vi "weather_station.vi"() -> ()   [LabVIEW 2023]
uses:
  <vilib>/Instr/_visa.llb/VISA Configure Serial Port (Instr).vi
  global_variables.vi
  <vilib>/addons/_JKI.lib/REST Client/classes/REST Client/REST Client.lvclass
  <vilib>/Analysis/NI_AALBase.lvlib
panel:
  in  "stop_button":bool
  in  "HELP_BUTTON":bool
  in  "SAVE DATA":bool
  in  "COUNT SERVER":i8 min=0
  in  "REQUEST_TO_SERVER":bool
  in  "LOAD_FROM_FILE":bool
  in  "PLAY_STOP_BUTTON":bool
  in  "ACQUISITION TIME":dbl min=0.0
  out "?":bool
  out "?":bool
  out "?":bool
  out "?":bool
  in  "VISA RESOURCE NAME":refnum<visa-resource-name>
  out "?":string[](array[string])
  out "?":string[](array[string])
  out "?":string[](array[string])
  out "HUMIDITY":dbl(knob) scale=0.0..100.0
  out "PERCEIVED TEMP.":dbl(slide) scale=0.0..100.0
  out "TEMPERATURE":dbl(slide) scale=0.0..100.0
  out "HUMIDITY TREND":cluster{dbl, dbl}(graph)
  out "PERCEIVED TEMP. TREND":cluster{dbl, dbl}(graph)
  out "TEMPERATURE TREND":cluster{dbl, dbl}(graph)
  # "ACQUISITION FROM ARDUINO"
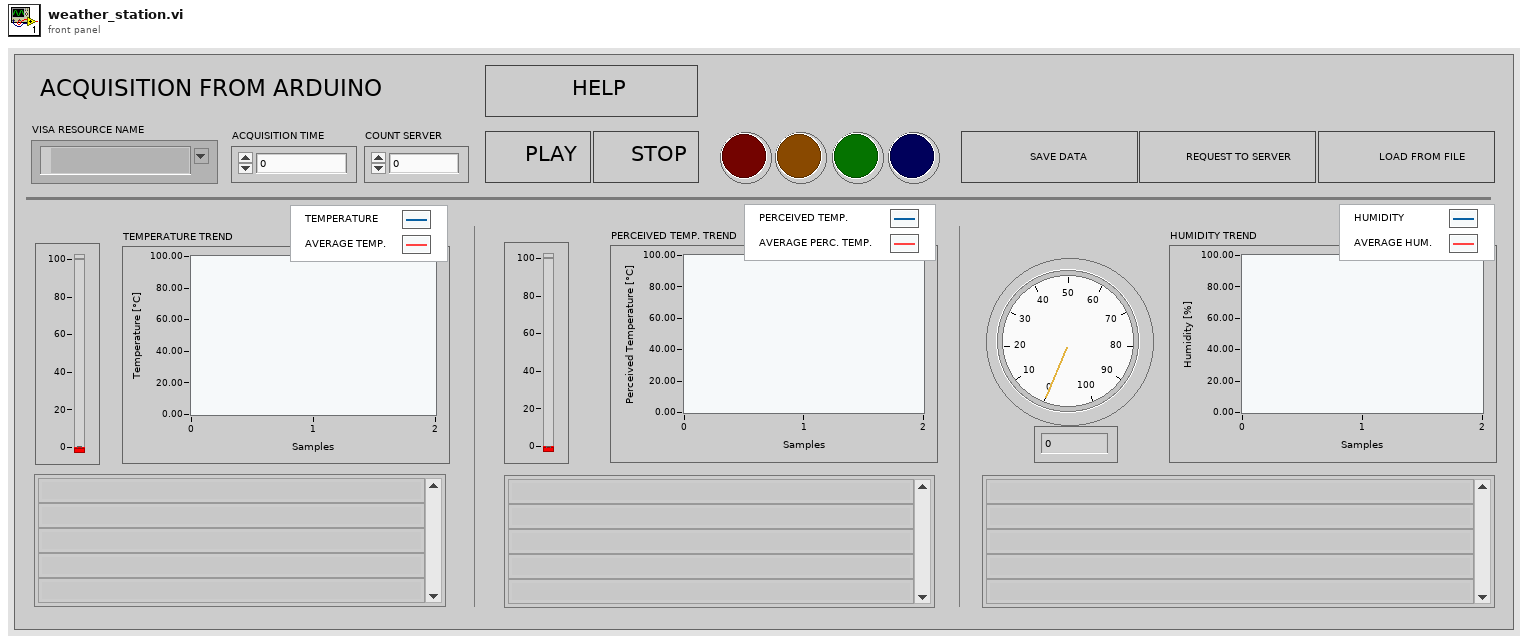
[diagram p1: front panel]
types:
  T1 = enum16{"open", "replace", "create", "open or create", "replace or create", "replace or create with confirmation"}
  T2 = enum32{"Invalid", "Standard", "Closed", "Hidden", "Minimized", "Maximized"}
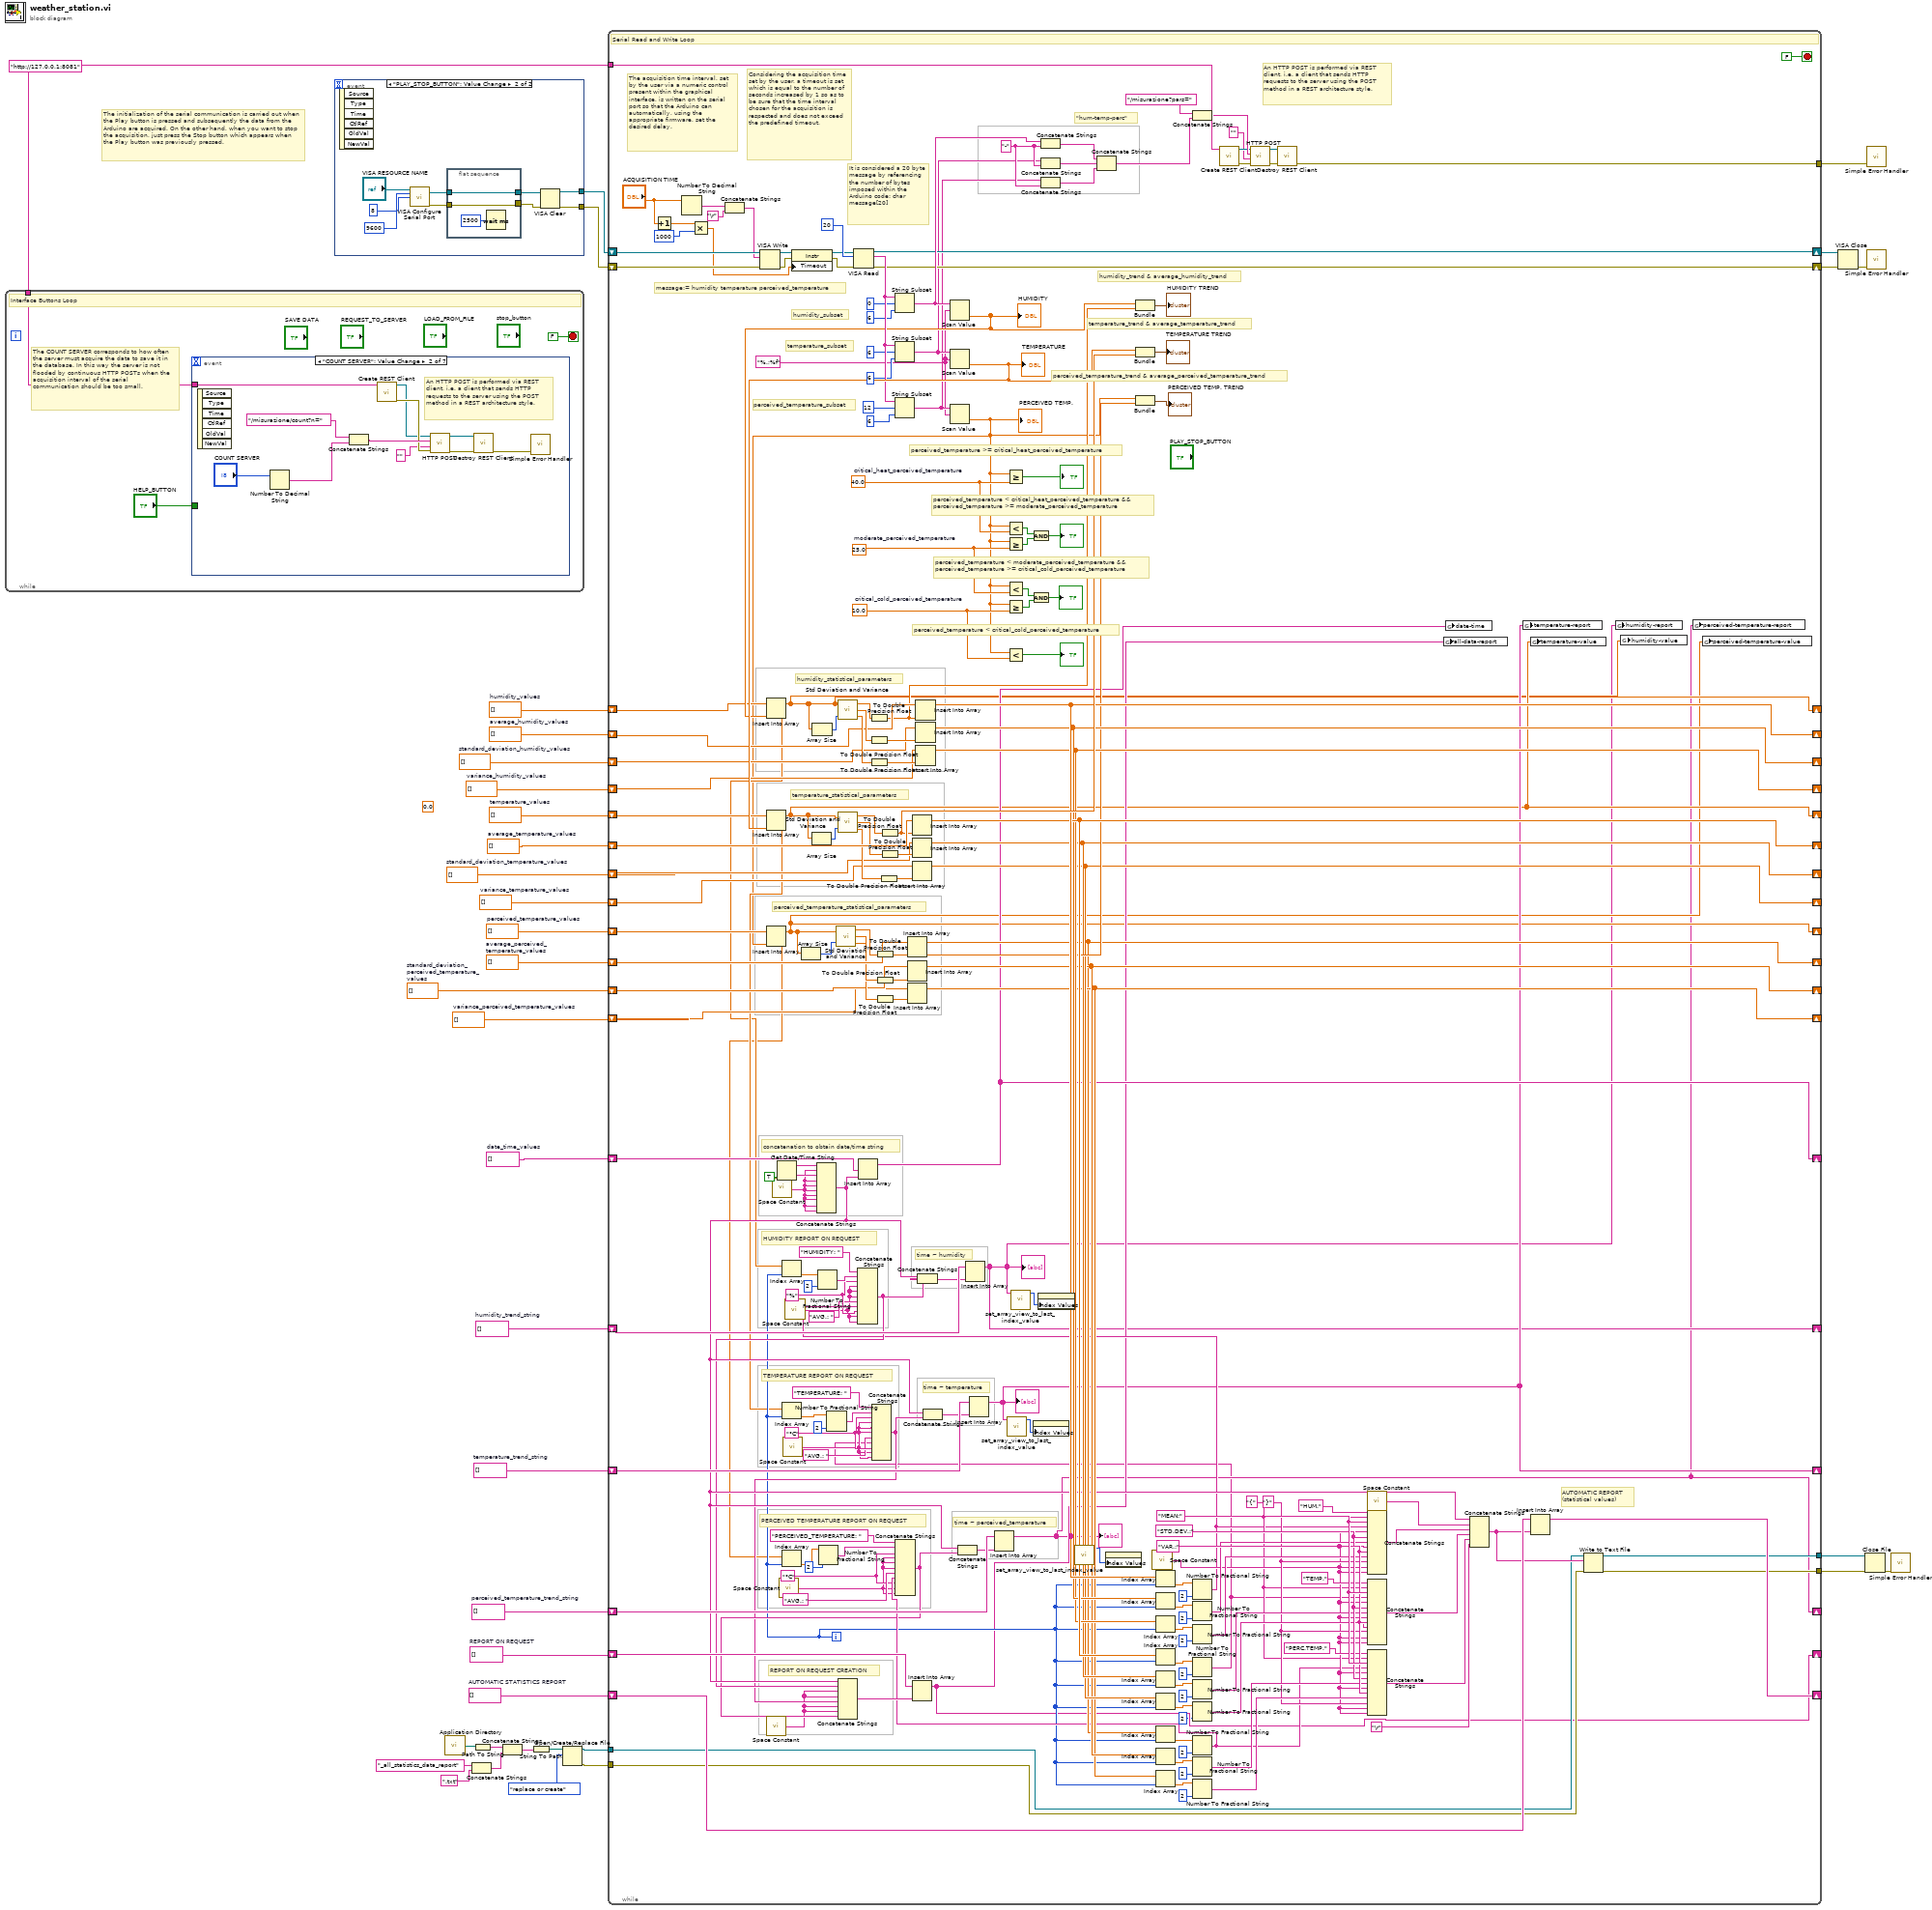
[diagram p0: block diagram]
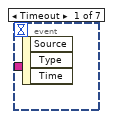
[diagram p2: hidden frame]
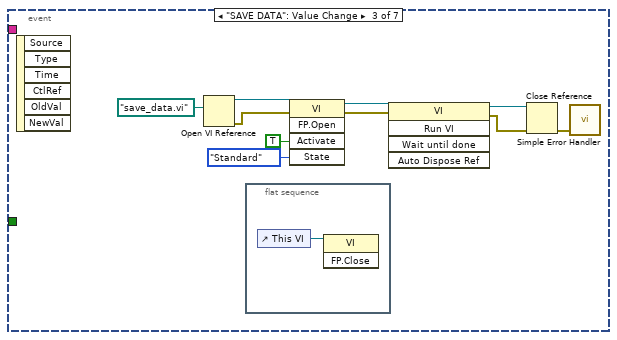
[diagram p3: hidden frame]
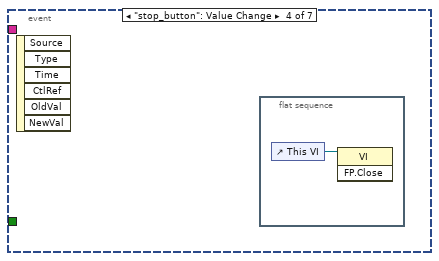
[diagram p4: hidden frame]
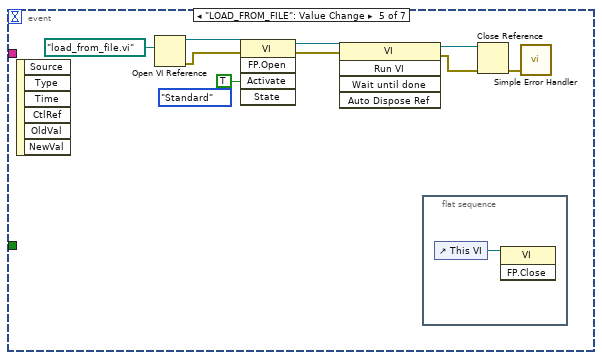
[diagram p5: hidden frame]
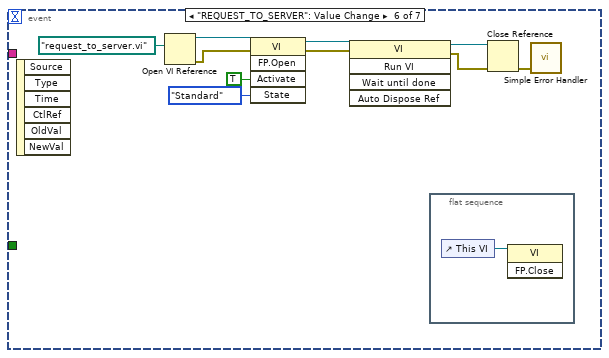
[diagram p6: hidden frame]
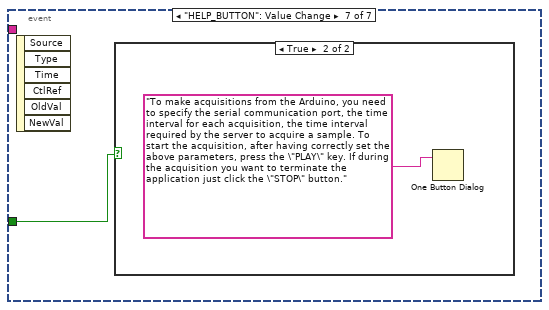
[diagram p7: hidden frame]
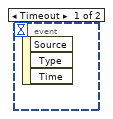
[diagram p9: hidden frame]
diagram:
  (unwired) 0.0
  w1 = "http://127.0.0.1:8081" ("Base URL")
  w18 = string[] []  # AUTOMATIC STATISTICS REPORT
  w19 = dbl[] []  # variance_perceived_temperature_values
  w20 = dbl[] []  # standard_deviation_perceived_temperature_values
  w21 = dbl[] []  # variance_temperature_values
  w22 = dbl[] []  # standard_deviation_temperature_values
  w23 = dbl[] []  # variance_humidity_values
  w24 = dbl[] []  # standard_deviation_humidity_values
  w28 = string[] []  # date_time_values
  w29 = dbl[] []  # average_perceived_temperature_values
  w30 = dbl[] []  # average_temperature_values
  w31 = dbl[] []  # average_humidity_values
  w32 = string[] []  # REPORT ON REQUEST
  w33 = string[] []  # perceived_temperature_trend_string
  w34 = string[] []  # temperature_trend_string
  w35 = string[] []  # humidity_trend_string
  w36 = dbl[] []  # perceived_temperature_values
  w37 = dbl[] []  # humidity_values
  w38 = dbl[] []  # temperature_values
  # "The initialization of the serial communication is carried out when the Play button is pressed and subsequently the data from the Arduino are acquired. On the other hand, when you want to stop the acquisition, just press the Stop button which appears when the Play button was previously pressed."
  n1 = while {
    tunnel: w1 -> [w40]
    stop <- FALSE stop-if-true
    # "The COUNT SERVER corresponds to how often the server must acquire the data to save it in the database. In this way the server is not flooded by continuous HTTP POSTs when the acquisition interval of the serial communication should be too small."
    # "Interface Buttons Loop"
    n2 = event shown="[1] \"COUNT SERVER\": Value Change" {
      selector: _ -> [_ _ _ _ _ _ _]
      dyn-events: _ -> [_ _ _ _ _ _ _]
      timeout: _ -> [_ _ _ _ _ _ _]
      tunnel: w40 -> [_ w44 _ _ _ _ _]
      tunnel: "HELP_BUTTON" -> [_ _ _ _ _ _ w86]
      event Timeout {
        n3 = event-data() -> ()  [unwired: 1 in, 3 out]
      }
      event "COUNT SERVER": Value Change {
        # "An HTTP POST is performed via REST client, i.e. a client that sends HTTP requests to the server using the POST method in a REST architecture style."
        n4 = event-data() -> ()  [unwired: 1 in, 6 out]
        n5 = Number To Decimal String(number="COUNT SERVER") -> (decimal integer string=w42:string)  [unwired: 1 in]
        n6 = Concatenate Strings("/misurazione/count?n=" ("Base URL"), w42) -> (w50:string)
        n7 = call <vilib>:"Create REST Client.vi"("Base URL"=w44) -> ("error out"=w49:errorcluster, "REST Client out"=w48:refnum<class "REST Client.lvclass">)  [unwired: 9 in]
        n8 = call-dynamic "HTTP POST.vi"("error in (no error)"=w49, "Request body"="", "Path"=w50, "REST Client in"=w48) -> ("error out"=w51:errorcluster, "REST Client out"=w52:refnum<class "REST Client.lvclass">)  [unwired: 2 in, 4 out]
        n9 = call-dynamic "Destroy REST Client.vi"("error in (no error)"=w51, "REST Client in"=w52) -> ("error out"=w45:errorcluster)  [unwired: 9 in]
        n10 = call <vilib>:"Simple Error Handler.vi"("error in (no error)"=w45) -> ()  [unwired: 4 in, 5 out]
      }
      event "SAVE DATA": Value Change {
        n11 = event-data() -> ()  [unwired: 1 in, 6 out]
        n12 = Open VI Reference(vi path=path "save_data.vi") -> (vi reference=w56:refnum<vi>, error out=w57:errorcluster)  [unwired: 5 in]
        n13 = flat-sequence {
          frame #0 {
            n14 = control-ref of="This VI"() -> (w63:refnum<vi>)
            n15 = invoke class="VI" method="FP.Close"(reference=w63) -> ()  [unwired: 2 in, 3 out]
          }
        }
        n16 = invoke class="VI" method="FP.Open"(reference=w56, error in=w57, "Activate"=TRUE ("Activate?"), "State"=T2."Standard") -> (reference out=w58:refnum<vi>, error out=w59:errorcluster)  [unwired: 1 in, 3 out]
        n17 = invoke class="VI" method="Run VI"(reference=w58, error in=w59) -> (reference out=w61:refnum<vi>, error out=w60:errorcluster)  [unwired: 3 in, 3 out]
        n18 = Close Reference(reference=w61, error in (no error)=w60) -> (error out=w62:errorcluster)
        n19 = call <vilib>:"Simple Error Handler.vi"("error in (no error)"=w62) -> ()  [unwired: 4 in, 5 out]
      }
      event "stop_button": Value Change {
        n20 = event-data() -> ()  [unwired: 1 in, 6 out]
        n21 = flat-sequence {
          frame #0 {
            n22 = control-ref of="This VI"() -> (w64:refnum<vi>)
            n23 = invoke class="VI" method="FP.Close"(reference=w64) -> ()  [unwired: 2 in, 3 out]
          }
        }
      }
      event "LOAD_FROM_FILE": Value Change {
        (unwired) T2."Standard" ("State")
        n24 = event-data() -> ()  [unwired: 1 in, 6 out]
        n25 = Open VI Reference(vi path=path "load_from_file.vi") -> (vi reference=w67:refnum<vi>, error out=w68:errorcluster)  [unwired: 5 in]
        n26 = invoke class="VI" method="FP.Open"(reference=w67, error in=w68, "Activate"=TRUE ("Activate?")) -> (reference out=w69:refnum<vi>, error out=w70:errorcluster)  [unwired: 2 in, 3 out]
        n27 = invoke class="VI" method="Run VI"(reference=w69, error in=w70) -> (reference out=w72:refnum<vi>, error out=w71:errorcluster)  [unwired: 3 in, 3 out]
        n28 = flat-sequence {
          frame #0 {
            n29 = control-ref of="This VI"() -> (w74:refnum<vi>)
            n30 = invoke class="VI" method="FP.Close"(reference=w74) -> ()  [unwired: 2 in, 3 out]
          }
        }
        n31 = Close Reference(reference=w72, error in (no error)=w71) -> (error out=w73:errorcluster)
        n32 = call <vilib>:"Simple Error Handler.vi"("error in (no error)"=w73) -> ()  [unwired: 4 in, 5 out]
      }
      event "REQUEST_TO_SERVER": Value Change {
        n33 = event-data() -> ()  [unwired: 1 in, 6 out]
        n34 = Open VI Reference(vi path=path "request_to_server.vi") -> (vi reference=w78:refnum<vi>, error out=w79:errorcluster)  [unwired: 5 in]
        n35 = invoke class="VI" method="FP.Open"(reference=w78, error in=w79, "Activate"=TRUE ("Activate?"), "State"=T2."Standard") -> (reference out=w80:refnum<vi>, error out=w81:errorcluster)  [unwired: 1 in, 3 out]
        n36 = invoke class="VI" method="Run VI"(reference=w80, error in=w81) -> (reference out=w83:refnum<vi>, error out=w82:errorcluster)  [unwired: 3 in, 3 out]
        n37 = flat-sequence {
          frame #0 {
            n38 = control-ref of="This VI"() -> (w85:refnum<vi>)
            n39 = invoke class="VI" method="FP.Close"(reference=w85) -> ()  [unwired: 2 in, 3 out]
          }
        }
        n40 = Close Reference(reference=w83, error in (no error)=w82) -> (error out=w84:errorcluster)
        n41 = call <vilib>:"Simple Error Handler.vi"("error in (no error)"=w84) -> ()  [unwired: 4 in, 5 out]
      }
      event "HELP_BUTTON": Value Change {
        n42 = event-data() -> ()  [unwired: 1 in, 6 out]
        n43 = case shown="True" w86 {
          frame False {
          }
          frame True {
            n44 = One Button Dialog(message="To make acquisitions from the Arduino, you need to specify the serial communication port, the time interval for each acquisition, the time interval required by the server to acquire a sample. To start the acquisition, after having correctly set the above parameters, press the \"PLAY\" key. If during the acquisition you want to terminate the application just click the \"STOP\" button.") -> ()  [unwired: 1 in, 1 out]
          }
        }
      }
    }
  }
  n45 = event shown="[1] \"PLAY_STOP_BUTTON\": Value Change" {
    selector: _ -> [_ _]
    dyn-events: _ -> [_ _]
    timeout: _ -> [_ _]
    tunnel: [_ w96] -> w3
    tunnel: [_ w95] -> w2
    event Timeout {
      n46 = event-data() -> ()  [unwired: 1 in, 3 out]
    }
    event "PLAY_STOP_BUTTON": Value Change {
      n47 = event-data() -> ()  [unwired: 1 in, 6 out]
      n48 = call-poly "VISA Configure Serial Port"("VISA resource name"="VISA RESOURCE NAME", "baud rate (9600)"=u32 9600, "data bits (8)"=u16 8) -> ("VISA resource name out"=w91:refnum<visa-resource-name>, "error out"=w92:errorcluster)  [unwired: 11 in]
      n49 = flat-sequence {
        tunnel: w91 -> [w98]
        tunnel: w92 -> [w97]
        tunnel: [w98] -> w93
        tunnel: [w97] -> w94
        frame #0 {
          n50 = Wait (ms)(milliseconds to wait=u32 2500) -> ()  [unwired: 1 out]
        }
      }
      n51 = VISA Clear(VISA resource name=w93, error in (no error)=w94) -> (VISA resource name out=w96:refnum<visa-resource-name>, error out=w95:errorcluster)
    }
  }
  n52 = call <vilib>:"Application Directory.vi"() -> ("Application Directory"=w10:path)
  n53 = Concatenate Strings("_all_statistics_data_report" ("string"), ".txt") -> (w14:string)
  n54 = Path To String(path=w10) -> (string=w11:string)
  n55 = Concatenate Strings(w11, w14) -> (w9:string)
  n56 = String To Path(string=w9) -> (path=w13:path)
  n57 = Open/Create/Replace File(file path (use dialog)=w13, operation (0:open)=T1."replace or create") -> (refnum out=w6:refnum<file>, error out=w5:errorcluster)  [unwired: 4 in, 1 out]
  n58 = while {
    shift-right: [w149] -> w27
    shift-left: w3 -> [w146]
    shift-right: [w148] -> w26
    shift-left: w2 -> [w145]
    shift-right: [w128] -> _
    shift-left: w38 -> [w282]
    shift-right: [w127] -> _
    shift-left: w37 -> [w242]
    shift-right: [w126] -> _
    shift-left: w36 -> [w281]
    shift-right: [w117] -> _
    shift-left: w35 -> [w265]
    shift-right: [w129] -> _
    shift-left: w34 -> [w263]
    shift-right: [w116] -> _
    shift-left: w33 -> [w261]
    shift-right: [w130] -> _
    shift-left: w32 -> [w259]
    shift-right: [w203] -> _
    shift-left: w31 -> [w244]
    shift-right: [w202] -> _
    shift-left: w30 -> [w268]
    shift-right: [w179] -> _
    shift-left: w29 -> [w252]
    shift-right: [w131] -> _
    shift-left: w28 -> [w257]
    shift-right: [w201] -> _
    shift-left: w24 -> [w241]
    shift-right: [w200] -> _
    shift-left: w23 -> [w240]
    shift-right: [w198] -> _
    shift-left: w22 -> [w234]
    shift-right: [w197] -> _
    shift-left: w21 -> [w233]
    shift-right: [w196] -> _
    shift-left: w20 -> [w225]
    shift-right: [w195] -> _
    shift-left: w19 -> [w224]
    shift-right: [w191] -> _
    shift-left: w18 -> [w190]
    tunnel: [w185] -> w8
    tunnel: [w184] -> w7
    tunnel: w6 -> [w159]
    tunnel: w5 -> [w183]
    tunnel: [w133] -> w4
    tunnel: w1 -> [w132]
    i -> [w155]
    stop <- FALSE stop-if-true
    w100 = "%.;%f" ("format string")
    w181 = "}"
    w175 = "{"
    w221 = "MEAN:"
    w220 = "VAR.:"
    w210 = "STD.DEV.:"
    w269 = "-" ("string")
    w167 = "°C"
    w171 = "°C"
    w173 = "%"
    w283 = 10.0  # critical_cold_perceived_temperature
    w288 = 25.0  # moderate_perceived_temperature
    w289 = 40.0  # critical_heat_perceived_temperature
    # "AUTOMATIC REPORT\n(statistical values)"
    # "An HTTP POST is performed via REST client, i.e. a client that sends HTTP requests to the server using the POST method in a REST architecture style."
    # "perceived_temperature_trend & average_perceived_temperature_trend"
    # "temperature_trend & average_temperature_trend"
    # "humidity_trend & average_humidity_trend"
    # "perceived_temperature_subset"
    # "temperature_subset"
    # "humidity_subset"
    # "The acquisition time interval, set by the user via a numeric control present within the graphical interface, is written on the serial port so that the Arduino can automatically, using the appropriate firmware, set the desired delay."
    # "Considering the acquisition time set by the user, a timeout is set which is equal to the number of seconds increased by 1 so as to be sure that the time interval chosen for the acquisition is respected and does not exceed the predefined timeout."
    # "perceived_temperature_statistical_parameters"
    # "temperature_statistical_parameters"
    # "humidity_statistical_parameters"
    # "REPORT ON REQUEST CREATION"
    # "\"hum-temp-perc\""
    # "time ~ perceived_temperature"
    # "time ~ temperature"
    # "time ~ humidity"
    # "PERCEIVED TEMPERATURE REPORT ON REQUEST"
    # "TEMPERATURE REPORT ON REQUEST"
    # "HUMIDITY REPORT ON REQUEST"
    # "concatenation to obtain date/time string"
    # "message:= humidity temperature perceived_temperature"
    # "perceived_temperature < critical_cold_perceived_temperature"
    # "perceived_temperature < moderate_perceived_temperature && perceived_temperature >= critical_cold_perceived_temperature"
    # "perceived_temperature < critical_heat_perceived_temperature && perceived_temperature >= moderate_perceived_temperature"
    # "perceived_temperature >= critical_heat_perceived_temperature"
    # "It is considered a 20 byte message by referencing the number of bytes imposed within the Arduino code: char message[20]"
    # "Serial Read and Write Loop"
    n59 = Increment(x="ACQUISITION TIME") -> (x+1=w139:dbl)
    n60 = Number To Decimal String(number="ACQUISITION TIME") -> (decimal integer string=w137:string)  [unwired: 1 in]
    n61 = Multiply(x=w139, y=i16 1000) -> (x*y=w142:dbl)
    n62 = Concatenate Strings(w137, "\r") -> (w136:string)
    n63 = VISA Write(VISA resource name=w146, write buffer=w136, error in (no error)=w145) -> (VISA resource name out=w144:refnum<visa-resource-name>, error out=w143:errorcluster)  [unwired: 1 out]
    n64 = call <vilib>:"Space Constant.vi"() -> ("String"=w161:string)
    n65 = call <vilib>:"Space Constant.vi"() -> ("String"=w160:string)
    n66 = Get Date/Time String(want seconds? (F)=TRUE) -> (date string=w267:string, time string=w266:string)  [unwired: 2 in]
    n67 = call <vilib>:"Space Constant.vi"() -> ("String"=w164:string)
    n68 = call <vilib>:"Space Constant.vi"() -> ("String"=w165:string)
    n69 = call <vilib>:"Space Constant.vi"() -> ("String"=w166:string)
    n70 = property class="Instr"(reference=w144, error in=w143, "Timeout"=w142) -> (reference out=w141:refnum<visa-resource-name>, error out=w140:errorcluster)
    n71 = Concatenate Strings(w267, w160, w266, w160, w160, w160, w160, w160, w160, w160) -> (w178:string)
    n72 = VISA Read(VISA resource name=w141, byte count=u32 20, error in (no error)=w140) -> (VISA resource name out=w149:refnum<visa-resource-name>, read buffer=w296:string, error out=w148:errorcluster)  [unwired: 1 out]
    n73 = Insert Into Array(array=w257, new element=w178) -> (w131:string[])  [unwired: 1 in]
    n74 = String Subset ("humidity_subset")(string=w296, offset (0)=0 ("offset"), length (rest)=6 ("default (0 I32)")) -> (substring=w298:string)
    n75 = String Subset ("temperature_subset")(string=w296, offset (0)=6 ("offset"), length (rest)=6 ("default (0 I32)")) -> (substring=w147:string)
    n76 = String Subset ("perceived_temperature_subset")(string=w296, offset (0)=12 ("offset"), length (rest)=6 ("default (0 I32)")) -> (substring=w102:string)
    n77 = Scan Value(string=w298, format string=w100) -> (value=w245:dbl)  [unwired: 1 in, 1 out]
    "HUMIDITY" <- w245
    n78 = Insert Into Array(array=w242, new element=w245) -> (w127:dbl[])  [unwired: 1 in]
    n79 = Index Array(array=w127, index=w155) -> (element=w256:dbl)
    n80 = Array Size(array=w127) -> (size(s)=w251:i32)
    n81 = Number To Fractional String(number=w256, precision (6)=i16 2) -> (F-format string=w223:string)  [unwired: 2 in]
    n82 = call <vilib>:"Std Deviation and Variance.vi"("X"=w127, "Weighting (Sample)"=w251) -> ("mean"=w250:dbl, "standard deviation"=w249:dbl, "variance"=w248:dbl)
    n83 = To Double Precision Float(number=w250) -> (double precision float=w243:dbl)
    n84 = To Double Precision Float(number=w249) -> (double precision float=w247:dbl)
    n85 = To Double Precision Float(number=w248) -> (double precision float=w246:dbl)
    n86 = Insert Into Array(array=w244, new element=w243) -> (w203:dbl[])  [unwired: 1 in]
    n87 = Insert Into Array(array=w241, new element=w247) -> (w201:dbl[])  [unwired: 1 in]
    n88 = Insert Into Array(array=w240, new element=w246) -> (w200:dbl[])  [unwired: 1 in]
    n89 = Scan Value(string=w147, format string=w100) -> (value=w299:dbl)  [unwired: 1 in, 1 out]
    "TEMPERATURE" <- w299
    n90 = Insert Into Array(array=w282, new element=w299) -> (w128:dbl[])  [unwired: 1 in]
    n91 = Index Array(array=w128, index=w155) -> (element=w255:dbl)
    n92 = Array Size(array=w128) -> (size(s)=w232:i32)
    n93 = Number To Fractional String(number=w255, precision (6)=i16 2) -> (F-format string=w274:string)  [unwired: 2 in]
    n94 = call <vilib>:"Std Deviation and Variance.vi"("X"=w128, "Weighting (Sample)"=w232) -> ("mean"=w239:dbl, "standard deviation"=w236:dbl, "variance"=w235:dbl)
    n95 = To Double Precision Float(number=w235) -> (double precision float=w237:dbl)
    n96 = To Double Precision Float(number=w239) -> (double precision float=w253:dbl)
    n97 = To Double Precision Float(number=w236) -> (double precision float=w238:dbl)
    n98 = Insert Into Array(array=w268, new element=w253) -> (w202:dbl[])  [unwired: 1 in]
    n99 = Insert Into Array(array=w234, new element=w238) -> (w198:dbl[])  [unwired: 1 in]
    n100 = Insert Into Array(array=w233, new element=w237) -> (w197:dbl[])  [unwired: 1 in]
    n101 = Scan Value(string=w102, format string=w100) -> (value=w101:dbl)  [unwired: 1 in, 1 out]
    "PERCEIVED TEMP." <- w101
    n102 = Insert Into Array(array=w281, new element=w101) -> (w126:dbl[])  [unwired: 1 in]
    n103 = Index Array(array=w126, index=w155) -> (element=w254:dbl)
    n104 = Array Size(array=w126) -> (size(s)=w231:i32)
    n105 = Number To Fractional String(number=w254, precision (6)=i16 2) -> (F-format string=w276:string)  [unwired: 2 in]
    n106 = call <vilib>:"Std Deviation and Variance.vi"("X"=w126, "Weighting (Sample)"=w231) -> ("mean"=w230:dbl, "standard deviation"=w229:dbl, "variance"=w228:dbl)
    n107 = To Double Precision Float(number=w230) -> (double precision float=w199:dbl)
    n108 = To Double Precision Float(number=w229) -> (double precision float=w226:dbl)
    n109 = To Double Precision Float(number=w228) -> (double precision float=w227:dbl)
    n110 = Insert Into Array(array=w252, new element=w199) -> (w179:dbl[])  [unwired: 1 in]
    n111 = Insert Into Array(array=w225, new element=w226) -> (w196:dbl[])  [unwired: 1 in]
    n112 = Insert Into Array(array=w224, new element=w227) -> (w195:dbl[])  [unwired: 1 in]
    n113 = Greater Or Equal?(x=w101, y=w289) -> (x >= y?=→"?":bool)
    n114 = Less?(x=w101, y=w289) -> (x < y?=w286:bool)
    n115 = Greater Or Equal?(x=w101, y=w288) -> (x >= y?=w287:bool)
    n116 = Less?(x=w101, y=w288) -> (x < y?=w285:bool)
    n117 = Greater Or Equal?(x=w101, y=w283) -> (x >= y?=w284:bool)
    n118 = Less?(x=w101, y=w283) -> (x < y?=→"?":bool)
    n119 = And(x=w286, y=w287) -> (x .and. y?=→"?":bool)
    n120 = And(x=w285, y=w284) -> (x .and. y?=→"?":bool)
    n121 = Concatenate Strings(w298, w269) -> (w270:string)
    n122 = Concatenate Strings(w147, w269) -> (w271:string)
    n123 = Concatenate Strings(w102, w269) -> (w272:string)
    n124 = Concatenate Strings(w270, w271, w272) -> (w134:string)
    n125 = Bundle(w245, w243) -> (→"HUMIDITY TREND":cluster{dbl, dbl})  [unwired: 1 in]
    n126 = Bundle(w299, w253) -> (→"TEMPERATURE TREND":cluster{dbl, dbl})  [unwired: 1 in]
    n127 = Bundle(w101, w199) -> (→"PERCEIVED TEMP. TREND":cluster{dbl, dbl})  [unwired: 1 in]
    n128 = call <vilib>:"Space Constant.vi"() -> ("String"=w177:string)
    n129 = Index Array(array=w203, index=w155) -> (element=w219:dbl)
    n130 = Index Array(array=w201, index=w155) -> (element=w218:dbl)
    n131 = Index Array(array=w200, index=w155) -> (element=w217:dbl)
    n132 = Index Array(array=w202, index=w155) -> (element=w216:dbl)
    n133 = Index Array(array=w198, index=w155) -> (element=w215:dbl)
    n134 = Index Array(array=w197, index=w155) -> (element=w214:dbl)
    n135 = Index Array(array=w179, index=w155) -> (element=w213:dbl)
    n136 = Index Array(array=w196, index=w155) -> (element=w212:dbl)
    n137 = Index Array(array=w195, index=w155) -> (element=w211:dbl)
    n138 = Number To Fractional String(number=w219, precision (6)=i16 2) -> (F-format string=w174:string)  [unwired: 2 in]
    n139 = Concatenate Strings("HUMIDITY: ", w223, w173, w166, w166, w166, "AVG.: ", w174, w173, w166, w166) -> (w176:string)
    n140 = Concatenate Strings(w178, w176) -> (w264:string)
    n141 = Insert Into Array(array=w265, new element=w264) -> (w117:string[])  [unwired: 1 in]
    "?" <- w117
    n142 = call "set_array_view_to_last_index_value.vi"("generic array trend_string"=w117) -> ("index"=w156:i32[])  [unwired: 10 in]
    n143 = property class="Arr (strict)"("Index Values"=w156) -> ()  [unwired: 2 in, 2 out]
    n144 = Number To Fractional String(number=w218, precision (6)=i16 2) -> (F-format string=w209:string)  [unwired: 2 in]
    n145 = Number To Fractional String(number=w217, precision (6)=i16 2) -> (F-format string=w208:string)  [unwired: 2 in]
    n146 = Number To Fractional String(number=w216, precision (6)=i16 2) -> (F-format string=w115:string)  [unwired: 2 in]
    n147 = Concatenate Strings("TEMPERATURE: ", w274, w171, w165, w165, w165, "AVG.: ", w115, w171, w165, w165) -> (w162:string)
    n148 = Concatenate Strings(w178, w162) -> (w262:string)
    n149 = Insert Into Array(array=w263, new element=w262) -> (w129:string[])  [unwired: 1 in]
    "?" <- w129
    n150 = call "set_array_view_to_last_index_value.vi"("generic array trend_string"=w129) -> ("index"=w158:i32[])  [unwired: 10 in]
    n151 = property class="Arr (strict)"("Index Values"=w158) -> ()  [unwired: 2 in, 2 out]
    n152 = Number To Fractional String(number=w215, precision (6)=i16 2) -> (F-format string=w207:string)  [unwired: 2 in]
    n153 = Number To Fractional String(number=w214, precision (6)=i16 2) -> (F-format string=w206:string)  [unwired: 2 in]
    n154 = Number To Fractional String(number=w213, precision (6)=i16 2) -> (F-format string=w168:string)  [unwired: 2 in]
    n155 = Concatenate Strings("PERCEIVED_TEMPERATURE: ", w276, w167, w164, w164, w164, "AVG.: ", w168, w167, w164, w164) -> (w163:string)
    n156 = Concatenate Strings(w178, w176, w161, w161, w162, w161, w161, w163) -> (w258:string)
    n157 = Insert Into Array(array=w259, new element=w258) -> (w130:string[])  [unwired: 1 in]
    n158 = Concatenate Strings(w178, w163) -> (w260:string)
    n159 = Insert Into Array(array=w261, new element=w260) -> (w116:string[])  [unwired: 1 in]
    "?" <- w116
    n160 = call "set_array_view_to_last_index_value.vi"("generic array trend_string"=w116) -> ("index"=w157:i32[])  [unwired: 10 in]
    n161 = property class="Arr (strict)"("Index Values"=w157) -> ()  [unwired: 2 in, 2 out]
    n162 = Number To Fractional String(number=w212, precision (6)=i16 2) -> (F-format string=w205:string)  [unwired: 2 in]
    n163 = Number To Fractional String(number=w211, precision (6)=i16 2) -> (F-format string=w204:string)  [unwired: 2 in]
    n164 = Concatenate Strings("/misurazione?pars=" ("Base URL"), w134) -> (w122:string)
    n165 = call <vilib>:"Create REST Client.vi"("Base URL"=w132) -> ("error out"=w121:errorcluster, "REST Client out"=w120:refnum<class "REST Client.lvclass">)  [unwired: 9 in]
    n166 = call-dynamic "HTTP POST.vi"("error in (no error)"=w121, "Request body"="", "Path"=w122, "REST Client in"=w120) -> ("error out"=w123:errorcluster, "REST Client out"=w124:refnum<class "REST Client.lvclass">)  [unwired: 2 in, 4 out]
    n167 = call-dynamic "Destroy REST Client.vi"("error in (no error)"=w123, "REST Client in"=w124) -> ("error out"=w133:errorcluster)  [unwired: 9 in]
    n168 = call <vilib>:"Space Constant.vi"() -> ("String"=w180:string)
    n169 = Concatenate Strings("HUM.", w175, w221, w174, w177, w210, w209, w177, w220, w208, w181, w177, w177) -> (w194:string)
    n170 = Concatenate Strings("TEMP.", w175, w221, w115, w177, w210, w207, w177, w220, w206, w181, w177, w177) -> (w193:string)
    n171 = Concatenate Strings("PERC.TEMP.", w175, w221, w168, w177, w210, w205, w177, w220, w204, w181, w177, w177) -> (w192:string)
    n172 = global write "global_variables.vi" "all-data-report"(w130) -> ()
    n173 = global write "global_variables.vi" "date-time"(w131) -> ()
    n174 = Concatenate Strings(w178, w180, w194, w193, w192, "\r") -> (w186:string)
    n175 = global write "global_variables.vi" "temperature-report"(w129) -> ()
    n176 = global write "global_variables.vi" "temperature-value"(w128) -> ()
    n177 = Insert Into Array(array=w190, new element=w186) -> (w191:string[])  [unwired: 1 in]
    n178 = Write to Text File(file (use dialog)=w159, text=w186, error in=w183) -> (refnum out=w185:refnum<file>, error out=w184:errorcluster)  [unwired: 1 in, 1 out]
    n179 = global write "global_variables.vi" "humidity-report"(w117) -> ()
    n180 = global write "global_variables.vi" "humidity-value"(w127) -> ()
    n181 = global write "global_variables.vi" "perceived-temperature-report"(w116) -> ()
    n182 = global write "global_variables.vi" "perceived-temperature-value"(w126) -> ()
  }
  n183 = VISA Close(VISA resource name=w27, error in (no error)=w26) -> (error out=w25:errorcluster)
  n184 = Close File(refnum=w8, error in=w7) -> (error out=w17:errorcluster)  [unwired: 1 out]
  n185 = call <vilib>:"Simple Error Handler.vi"("error in (no error)"=w4) -> ()  [unwired: 4 in, 5 out]
  n186 = call <vilib>:"Simple Error Handler.vi"("error in (no error)"=w25) -> ()  [unwired: 4 in, 5 out]
  n187 = call <vilib>:"Simple Error Handler.vi"("error in (no error)"=w17) -> ()  [unwired: 4 in, 5 out]
